vi "Get XRS450 YAW.vi"(1 "Reset Angle?":bool) -> (0 "Angle":dbl(knob) scale=0.0..360.0)   [LabVIEW 2015]
uses:
  <vilib>/Rock Robotics/Network Tables/SD Write Boolean.vi
panel:
  out "Calibrated?":bool
  out "Device Found":bool
  # "Set these inputs before running."
  # "This can be set while running."
  # "This will display the current gyro angle."
  # "This shows wiring for the Analog Devices XRS450 gyro.  It can be plugged directly into the SPI port."
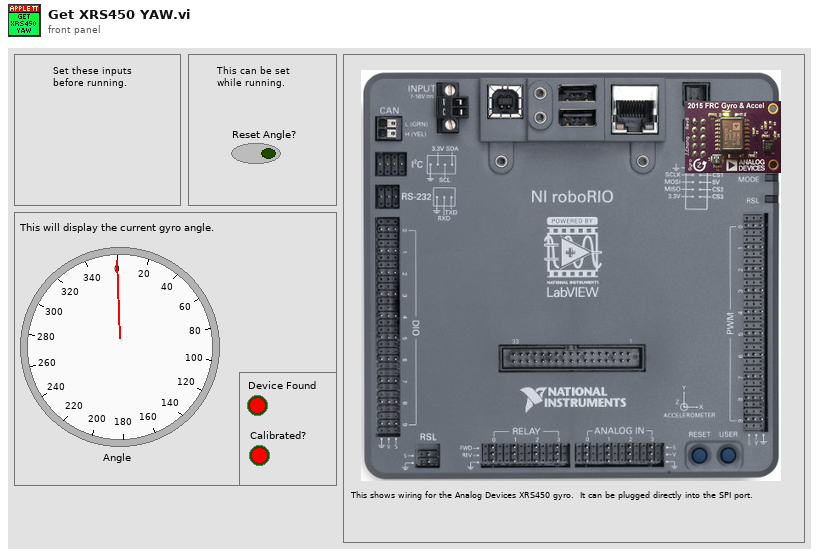
[diagram p1: front panel]
types:
  T1 = typedef "WPI_GyroDevRef.ctl" = cluster{"DevStatus":errorcluster, "Analog Channel":T2, "Offset":dbl, "Gain (VoltsPerDegree/Second)":dbl, "Gyro Type":enum16{"Analog", "XRS450"}, "Handle":i32, "SPI Bus":T3, "Device Found":bool, "Sample Rate":dbl, "Calibrate On Open":bool}
  T2 = typedef "FPGA_AIChannel.ctl" = enum8{"AI 0", "AI 1", "AI 2", "AI 3", "AI MXP 0", "AI MXP 1", "AI MXP 2", "AI MXP 3", "Invalid"}
  T3 = typedef "spi_bus.ctl" = enum16{"SPI On-Board, CS0", "SPI On-Board, CS1", "SPI On-Board, CS2", "SPI On-Board, CS3", "SPI MXP", "Invalid"}
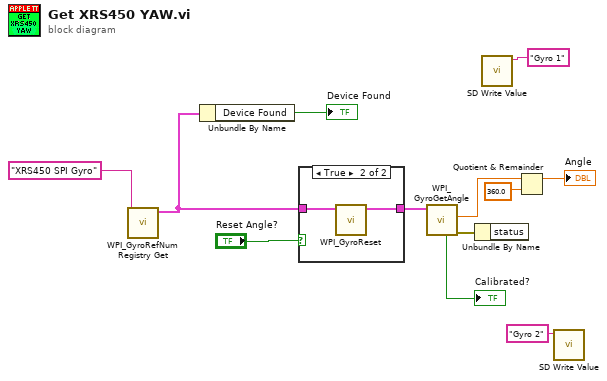
[diagram p0: block diagram]
diagram:
  n1 = call <vilib>:"WPI_GyroRefNum Registry Get.vi"("refnum name"="XRS450 SPI Gyro") -> ("GyroDevRef"=w9:T1)  [unwired: 9 in, 1 out]
  n2 = Unbundle By Name(w9) -> ("Device Found"=→"Device Found":bool)
  n3 = case shown="True" "Reset Angle?" {
    tunnel: w9 -> [w13 w15]
    tunnel: [w13 w14] -> w6
    frame False {
    }
    frame True {
      n4 = call <vilib>:"WPI_GyroReset.vi"("GyroDevRef"=w15) -> ("GyroDevRef"=w14:T1)  [unwired: 9 in, 1 out]
    }
  }
  n5 = call <vilib>:"WPI_GyroGetAngle.vi"("GyroDevRef"=w6) -> ("error out"=w4:errorcluster, "Angle"=w5:dbl, "Calibrated?"=→"Calibrated?":bool)  [unwired: 6 in, 2 out]
  n6 = Unbundle By Name(w4) -> ()  [unwired: 1 out]
  n7 = call-poly <vilib>:"SD Write Value.vi"("Name"="Gyro 1") -> ()  [unwired: 9 in, 2 out]
  n8 = Quotient & Remainder(x=w5, y=360.0) -> (x-y*floor(x/y)=→"Angle":dbl)  [unwired: 1 out]
  n9 = call-poly <vilib>:"SD Write Value.vi"("Name"="Gyro 2") -> ()  [unwired: 9 in, 2 out]
